vi "POP_Lookup.vi"(7 "Name":string, 8 "error in (no error)":errorcluster, 9 "Point":cluster{"X":i32, "Y":i32}, 11 "Ctl Refnum":refnum<vi>) -> (0 "error out":errorcluster, 1 "In Bounds?":bool, 2 "Found":bool, 3 "Popup Parameters":T3={"Prop Type"=enum."Unkown", "Initial Value"=variant, "Caption Strings"=[], "Ring Strings"=[], "Cell Rect"={"left"=0, "top"=0, "right"=0, "bottom"=0}, "Mouse Coords"={"x"=0, "y"=0}, "Call Data"=variant, "Ring Values"=[], "Browse Options"={"Prompt"="", "Match Pattern"="", "Mode"=enum."existing file", "Start Path"=path "", "Pattern Label"="", "Button Text"=""}, "Combo Box"={"Allow Undefined Strings"=FALSE}}, 4 "Cell Info (Call data)":T1={"Tag"="", "Row"=0, "Column"=0, "In Symbol?"=FALSE, "In Data?"=FALSE, "Cell String"="", "Ctl Refnum"=refnum, "Prop Type"=enum."Unkown", "Ring Strings"=[], "Ring Values"=[], "New Cell String"=""})   [LabVIEW 2016]
uses:
  Private/Ctrls/POP_Popup Call Parameters.ctl
  Private/Ctrls/POP_Data Type.ctl
  <vilib>/Utility/miscctls.llb/LVBrowseOptionsTypeDef.ctl
  Private/Ctrls/PSPOP_Grid.Cell Info.ctl
  Private/Ctrls/POP_Popup Operation.ctl
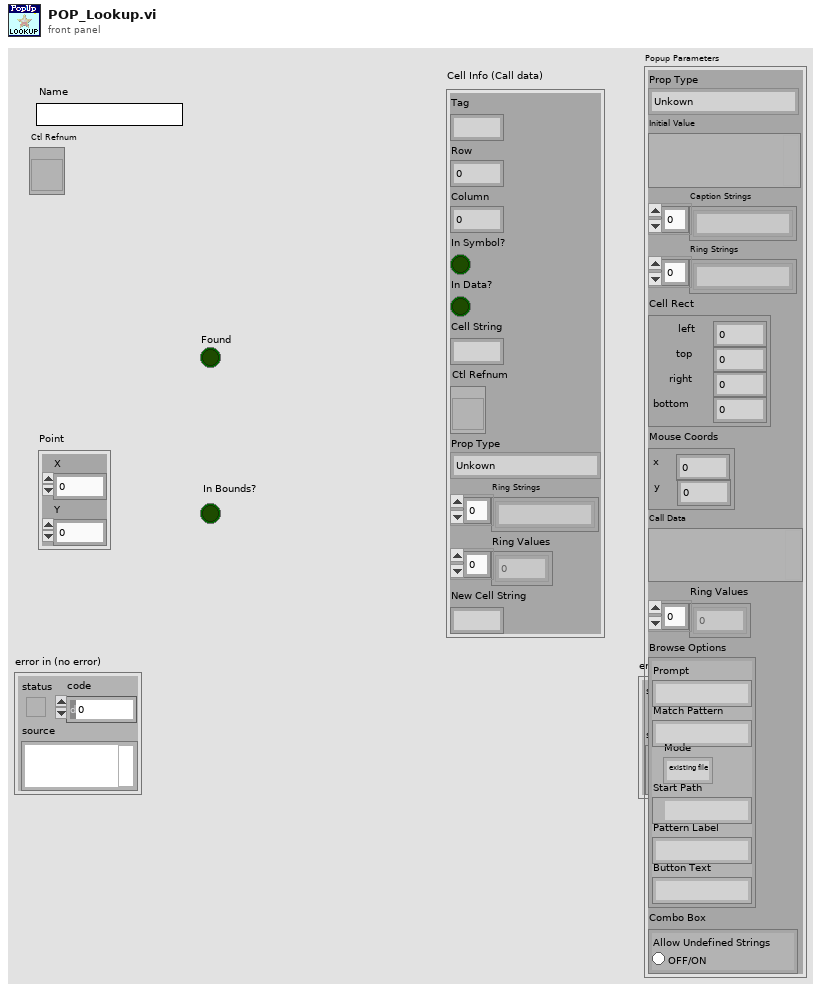
[diagram p1: front panel]
types:
  T1 = typedef "PSPOP_Grid.Cell Info.ctl" = cluster{"Tag":string, "Row":i32, "Column":i32, "In Symbol?":bool, "In Data?":bool, "Cell String":string, "Ctl Refnum":refnum<vi>, "Prop Type":T2, "Ring Strings":string[], "Ring Values":ext[], "New Cell String":string}
  T2 = typedef "POP_Data Type.ctl" = enum16{"NO POPUP", "Unkown", "String", "Integer", "Float", "Color", "Boolean", "Ring", "Captioned String", "Captioned Integer", "Button Color", "2 Int Cluster", "4 Int Cluster", "6-Dbl Cluster", "Path", "Combox", "Time", "ShotCut String"}
  T3 = typedef "POP_Popup Call Parameters.ctl" = cluster{"Prop Type":T2, "Initial Value":variant, "Caption Strings":string[], "Ring Strings":string[], "Cell Rect":cluster{"left":i16, "top":i16, "right":i16, "bottom":i16}, "Mouse Coords":cluster{"x":i16, "y":i16}, "Call Data":variant, "Ring Values":ext[], "Browse Options":T4, "Combo Box":cluster{"Allow Undefined Strings":bool}}
  T4 = typedef "LVBrowseOptionsTypeDef.ctl" = cluster{"Prompt":string, "Match Pattern":string, "Mode":enum32{"existing file", "new file", "new or existing file", "existing dir", "new dir", "new or existing dir", "existing file (use LLBs)", "new file (use LLBs)", "new or existing file (use LLBs)", "new or existing file or directory (use LLBs)", "existing dir (use LLBs)", "new dir (use LLBs)", "new or existing dir (use LLBs)", "existing file or dir", "new file or dir", "new or existing file or dir", "existing file or dir (use LLBs)", "new file or dir (use LLBs)"}, "Start Path":path, "Pattern Label":string, "Button Text":string}
  T5 = typedef "POP_Popup Operation.ctl" = enum16{"Show", "Initialize", "Close", "Popup Done", "Register a Location's Type", "Retrieve Location's Type"}
  T6 = cluster{"left":i16, "top":i16, "right":i16, "bottom":i16}
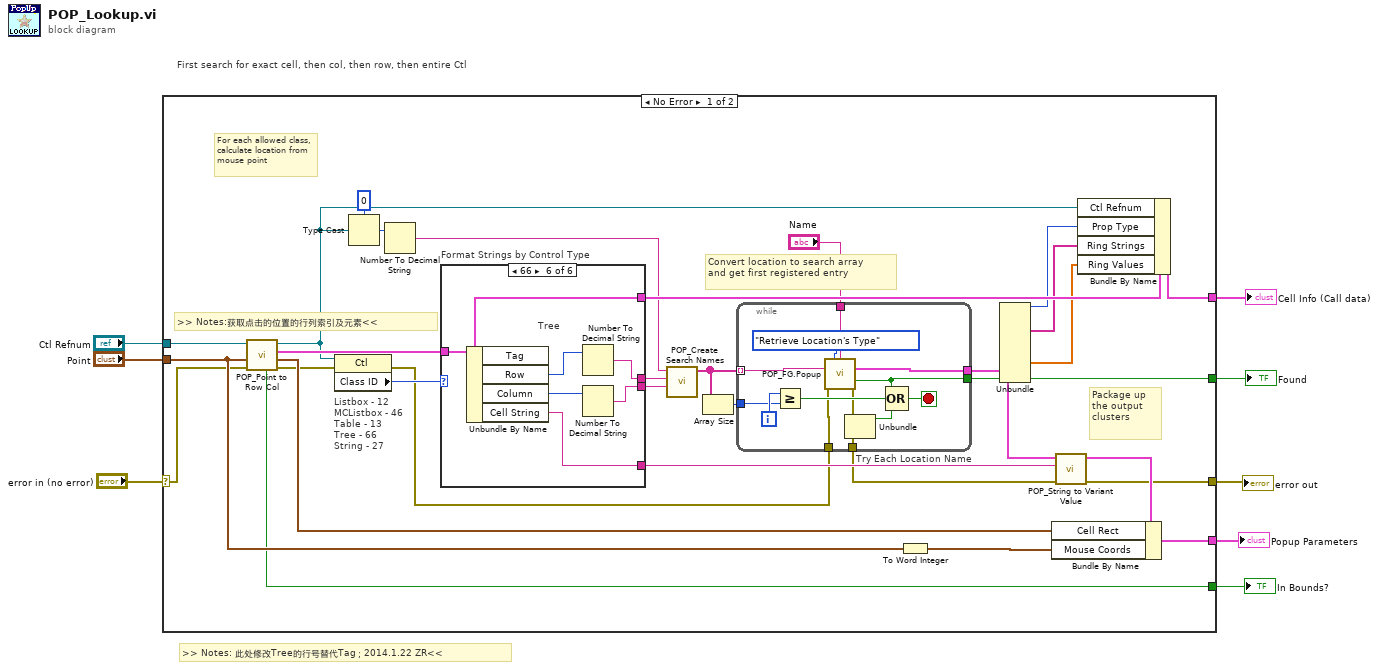
[diagram p0: block diagram]
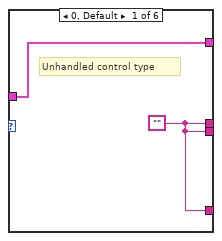
[diagram p2: hidden frame]
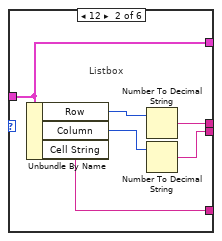
[diagram p3: hidden frame]
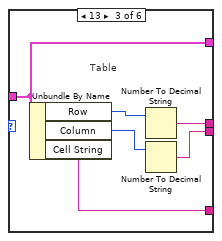
[diagram p4: hidden frame]
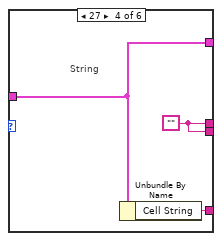
[diagram p5: hidden frame]
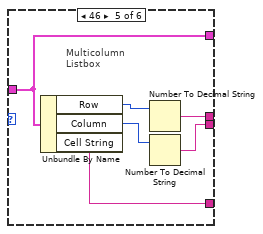
[diagram p6: hidden frame]
diagram:
  # ">> Notes: 此处修改Tree的行号替代Tag；2014.1.22 ZR<<"
  # "First search for exact cell, then col, then row, then entire Ctl"
  n1 = case shown="No Error" "error in (no error)" {
    selector: "error in (no error)" -> [w11 w81]
    tunnel: [w21 w81] -> w6
    tunnel: "Ctl Refnum" -> [w20 _]
    tunnel: "Point" -> [w18 _]
    tunnel: [w34 _] -> w7
    tunnel: [w29 _] -> w5
    tunnel: [w15 _] -> w4
    tunnel: [w27 _] -> w8
    frame No Error {
      # ">> Notes:获取点击的位置的行列索引及元素<<"
      # "Package up\nthe output\nclusters"
      # "Convert location to search array\nand get first registered entry"
      # "For each allowed class,\ncalculate location from\nmouse point"
      # "Listbox - 12\nMCListbox - 46\nTable - 13\nTree - 66\nString - 27"
      n2 = call "POP_Point to Row Col.vi"("error in (no error)"=w11, "Point"=w18, "Grid Ctl Reference In"=w20) -> ("error out"=w14:errorcluster, "Cell Rect Out"=w17:T6, "Cell Info Out"=w19:T1, "Grid Ctl Reference Out"=w12:refnum<vi>, "In Bounds?"=w15:bool)  [unwired: 4 in]
      n3 = property class="Ctl"(reference=w12, error in=w14) -> (error out=w13:errorcluster, "Class ID"=w39:u32)  [unwired: 1 out]
      n4 = Type Cast(type=0, x=w12) -> (*(type *) &x=w37:i32)
      n5 = Number To Decimal String(number=w37) -> (decimal integer string=w16:string)  [unwired: 1 in]
      n6 = case "Format Strings by Control Type" shown="66" w39 {
        tunnel: [w53 w58 w64 w68 w73 w76] -> w33
        tunnel: [w53 w56 w63 w68 w72 w79] -> w32
        tunnel: [w53 w55 w65 w67 w74 w78] -> w28
        tunnel: [w52 w54 w60 w66 w69 w77] -> w26
        tunnel: w19 -> [w52 w54 w60 w66 w69 w77]
        frame 0, Default {
          w53 = ""
          # "Unhandled control type"
        }
        frame 12 {
          # "Listbox"
          n7 = Unbundle By Name(w54) -> ("Row"=w59:i32, "Column"=w57:i32, "Cell String"=w55:string)
          n8 = Number To Decimal String(number=w59) -> (decimal integer string=w58:string)  [unwired: 1 in]
          n9 = Number To Decimal String(number=w57) -> (decimal integer string=w56:string)  [unwired: 1 in]
        }
        frame 13 {
          # "Table"
          n10 = Unbundle By Name(w60) -> ("Row"=w62:i32, "Column"=w61:i32, "Cell String"=w65:string)
          n11 = Number To Decimal String(number=w62) -> (decimal integer string=w64:string)  [unwired: 1 in]
          n12 = Number To Decimal String(number=w61) -> (decimal integer string=w63:string)  [unwired: 1 in]
        }
        frame 27 {
          w68 = ""
          # "String"
          n13 = Unbundle By Name(w66) -> ("Cell String"=w67:string)
        }
        frame 46 {
          # "Multicolumn\nListbox"
          n14 = Unbundle By Name(w69) -> ("Row"=w71:i32, "Column"=w70:i32, "Cell String"=w74:string)
          n15 = Number To Decimal String(number=w71) -> (decimal integer string=w73:string)  [unwired: 1 in]
          n16 = Number To Decimal String(number=w70) -> (decimal integer string=w72:string)  [unwired: 1 in]
        }
        frame 66 {
          # "Tree"
          n17 = Unbundle By Name(w77) -> ("Row"=w75:i32, "Column"=w80:i32, "Cell String"=w78:string)  [unwired: 1 out]
          n18 = Number To Decimal String(number=w75) -> (decimal integer string=w76:string)  [unwired: 1 in]
          n19 = Number To Decimal String(number=w80) -> (decimal integer string=w79:string)  [unwired: 1 in]
        }
      }
      n20 = call "POP_Create Search Names.vi"("Column String"=w32, "Tag or Row String"=w33, "Control Ref String"=w16) -> ("Search Names"=w36:string[])  [unwired: 8 in]
      n21 = Array Size(array=w36) -> (size(s)=w35:i32)
      n22 = while "Try Each Location Name" {
        tunnel: [w51] -> w25
        tunnel: w36 -> [w49] mode=indexing
        tunnel: w35 -> [w47]
        tunnel: [w45] -> w34
        tunnel: w13 -> [w42]
        tunnel: [w41] -> w22
        tunnel: "Name" -> [w40]
        i -> [w48]
        stop <- w43 stop-if-true
        n23 = Greater Or Equal?(x=w48, y=w47) -> (x >= y?=w46:bool)
        n24 = call "POP_FG.Popup.vi"("Popup Operation"=POP_Popup_Operation."Retrieve Location's Type", "Name"=w40, "Encoded Location"=w49, "Error In"=w42) -> ("Popup Parameters out"=w51:T3, "Found"=w45:bool, "Error Out"=w41:errorcluster)  [unwired: 8 in, 1 out]
        n25 = Unbundle(w41) -> ("status"=w44:bool)  [unwired: 2 out]
        n26 = Compound Arithmetic op=OR(w45, w46, w44) -> (w43:bool)
      }
      n27 = To Word Integer(number=w18) -> (16bit integer=w31:cluster{"X":i16, "Y":i16})
      n28 = Unbundle(w25) -> ("Prop Type"=w23:T2, "Ring Strings"=w24:string[], "Ring Values"=w9:ext[])  [unwired: 7 out]
      n29 = call "POP_String to Variant Value.vi"("error in (no error)"=w22, "Cell String"=w28, "Popup Parameters"=w25) -> ("error out"=w21:errorcluster, "Popup Parameters out"=w30:T3)  [unwired: 6 in, 1 out]
      n30 = Bundle By Name(cluster=w30, "Cell Rect"=w17, "Mouse Coords"=w31) -> (w29:T3)
      n31 = Bundle By Name(cluster=w26, "Ctl Refnum"=w12, "Prop Type"=w23, "Ring Strings"=w24, "Ring Values"=w9) -> (w27:T1)
    }
    frame Error {
    }
  }
  "error out" <- w6
  "Found" <- w7
  "In Bounds?" <- w4
  "Popup Parameters" <- w5
  "Cell Info (Call data)" <- w8
